vi "RFswitch2.vi"() -> ()   [LabVIEW 2013]
uses:
  Global 1.vi
panel:
  out "Ping result":u8 format="%x"
  out "Status":i32=1
  in  "RF Channel":u32=4 min=1 max=4 step=1
  out "Bytes Written 6":i32=5
  out "Bytes Read 6":i32
  out "Read Array 6":i32[](array[numeric])
  out "Write Array 6":i32[](array[numeric])=[5, 53, 6, 0, 0]
  out "Bytes Written 7":i32=5
  out "Bytes Read 7":i32
  out "Read Array 7":i32[](array[numeric])
  out "Write Array 7":i32[](array[numeric])=[5, 53, 7, 0, 0]
  out "Handle":u32=263961288
  in  "Controller Device Description":string="DLP-IO20"
  # "RF switch control panel"
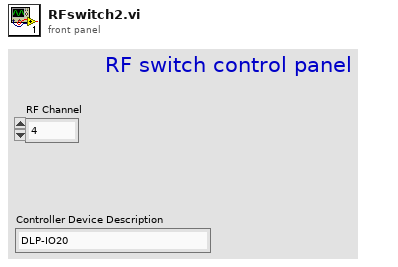
[diagram p1: front panel]
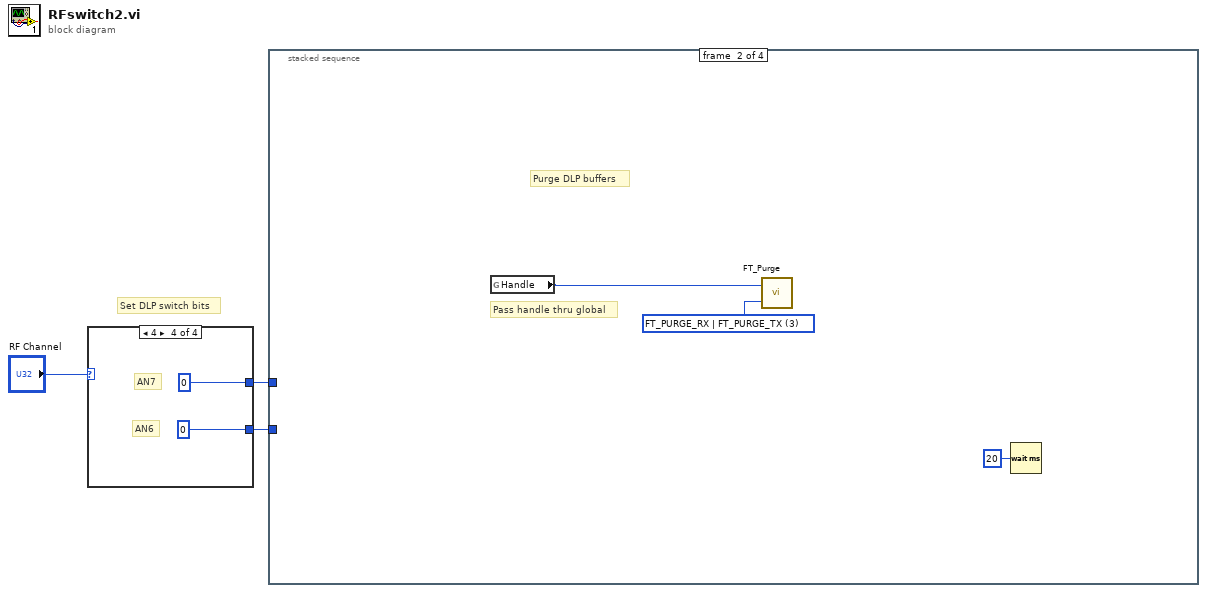
[diagram p0: block diagram]
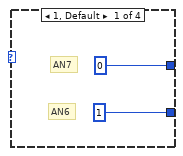
[diagram p2: hidden frame]
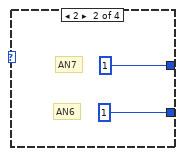
[diagram p3: hidden frame]
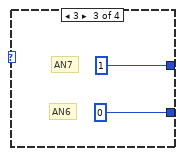
[diagram p4: hidden frame]
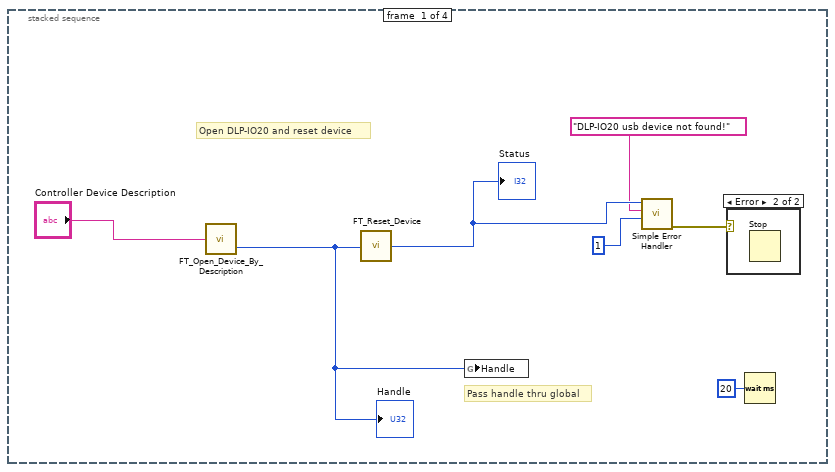
[diagram p5: hidden frame]
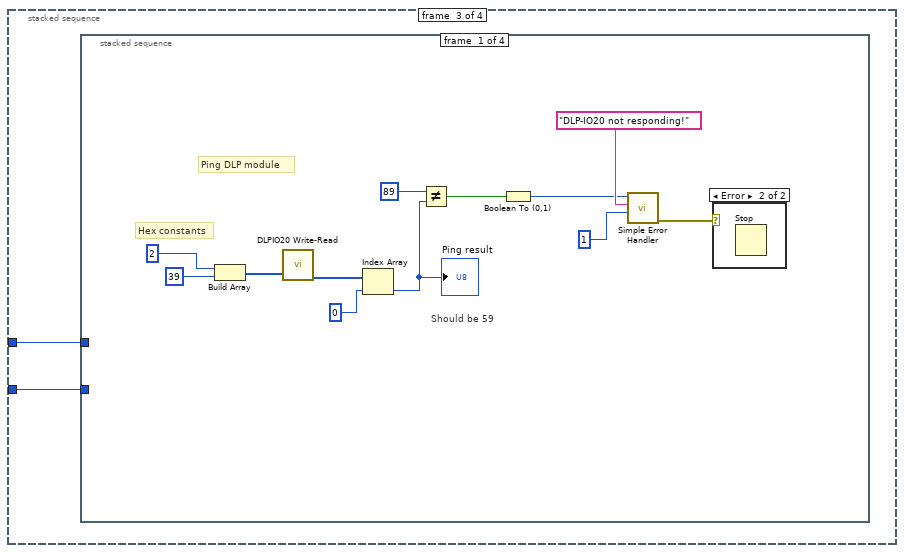
[diagram p7: hidden frame]
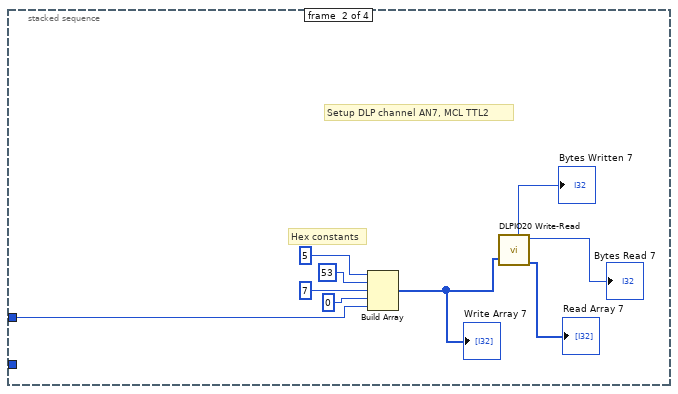
[diagram p9: hidden frame]
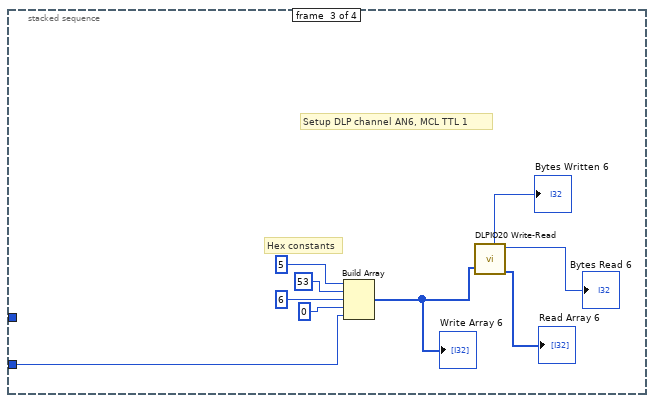
[diagram p10: hidden frame]
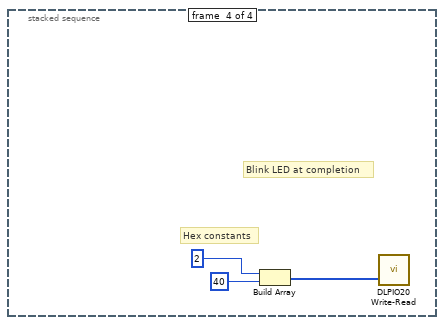
[diagram p11: hidden frame]
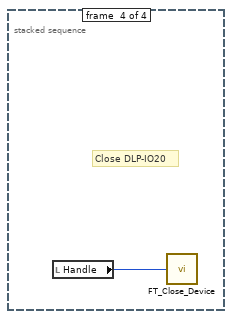
[diagram p12: hidden frame]
diagram:
  # "Set DLP switch bits"
  n1 = case shown="4" "RF Channel" {
    tunnel: [0 1 1 0] -> w2
    tunnel: [1 1 0 0] -> w1
    frame 1, Default {
      # "AN6"
      # "AN7"
    }
    frame 2 {
      # "AN6"
      # "AN7"
    }
    frame 3 {
      # "AN6"
      # "AN7"
    }
    frame 4 {
      # "AN6"
      # "AN7"
    }
  }
  n2 = stacked-sequence {
    tunnel: w2 -> [_ _ w23 _]
    tunnel: w1 -> [_ _ w22 _]
    frame #0 {
      # "Pass handle thru global"
      # "Open DLP-IO20 and reset device"
      n3 = call "FT_Open_Device_By_Description.vi"("Device Description"="Controller Device Description") -> ("Handle"=w16:u32)  [unwired: 1 out]
      "Handle" <- w16
      n4 = call "FT_Reset_Device.vi"("Handle"=w16) -> ("FT_Status"=w15:u32)
      "Status" <- w15
      n5 = global write "Global 1.vi" "Handle"(w16) -> ()
      n6 = call <vilib>:"Simple Error Handler.vi"("error code (no error:0)"=w15, "error source (\" \")"="DLP-IO20 usb device not found!", "type of dialog (OK msg:1)"=1) -> ("error out"=w12:errorcluster)  [unwired: 2 in, 4 out]
      n7 = case shown="Error" w12 {
        frame No Error {
        }
        frame Error {
          n8 = Stop() -> ()  [unwired: 1 in]
        }
      }
      n9 = Wait (ms)(milliseconds to wait=u32 20) -> ()  [unwired: 1 out]
    }
    frame #1 {
      w21 = u32 3 items=["FT_PURGE_RX"=1, "FT_PURGE_TX"=2, "FT_PURGE_RX | FT_PURGE_TX"=3] ("Purge Flags")
      # "Purge DLP buffers"
      # "Pass handle thru global"
      n10 = global read "Global 1.vi" "Handle"() -> (w20:u32)
      n11 = call "FT_Purge.vi"("Purge Flags"=w21, "Handle"=w20) -> ()  [unwired: 1 out]
      n12 = Wait (ms)(milliseconds to wait=u32 20) -> ()  [unwired: 1 out]
    }
    frame #2 {
      n13 = stacked-sequence {
        tunnel: w23 -> [_ w36 _ _]
        tunnel: w22 -> [_ _ w45 _]
        frame #0 {
          # "Should be 59"
          # "Ping DLP module"
          # "Hex constants"
          n14 = Build Array "Build Array"(u8 2, u8 39) -> (w33:u8[])
          n15 = call "DLPIO20 Write-Read.vi"("Write Buffer"=w33) -> ("Read Buffer Out"=w32:u8[])  [unwired: 3 in, 2 out]
          n16 = Index Array(array=w32, index=u8 0) -> (element=w29:u8)
          "Ping result" <- w29
          n17 = Not Equal?(x=u8 89, y=w29) -> (x != y?=w25:bool)
          n18 = Boolean To (0,1)(Boolean=w25) -> (0, 1=w24:i16)
          n19 = call <vilib>:"Simple Error Handler.vi"("error code (no error:0)"=w24, "error source (\" \")"="DLP-IO20 not responding!", "type of dialog (OK msg:1)"=1) -> ("error out"=w26:errorcluster)  [unwired: 2 in, 4 out]
          n20 = case shown="Error" w26 {
            frame No Error {
            }
            frame Error {
              n21 = Stop() -> ()  [unwired: 1 in]
            }
          }
        }
        frame #1 {
          # "Setup DLP channel AN7, MCL TTL2"
          # "Hex constants"
          n22 = Build Array "Build Array"(u8 5, u8 53, u8 7, u8 0, w36) -> (w39:i32[])
          "Write Array 7" <- w39
          n23 = call "DLPIO20 Write-Read.vi"("Write Buffer"=w39) -> ("Read Buffer Out"=→"Read Array 7":u8[], "Bytes Read"=→"Bytes Read 7":u32, "Bytes Written"=→"Bytes Written 7":u32)  [unwired: 3 in]
        }
        frame #2 {
          # "Setup DLP channel AN6, MCL TTL 1"
          # "Hex constants"
          n24 = Build Array "Build Array"(u8 5, u8 53, u8 6, u8 0, w45) -> (w48:i32[])
          "Write Array 6" <- w48
          n25 = call "DLPIO20 Write-Read.vi"("Write Buffer"=w48) -> ("Read Buffer Out"=→"Read Array 6":u8[], "Bytes Read"=→"Bytes Read 6":u32, "Bytes Written"=→"Bytes Written 6":u32)  [unwired: 3 in]
        }
        frame #3 {
          # "Blink LED at completion"
          # "Hex constants"
          n26 = Build Array "Build Array"(u8 2, u8 40) -> (w54:u8[])
          n27 = call "DLPIO20 Write-Read.vi"("Write Buffer"=w54) -> ()  [unwired: 3 in, 3 out]
        }
      }
    }
    frame #3 {
      # "Close DLP-IO20"
      n28 = local read "Handle"() -> (w57:u32)
      n29 = call "FT_Close_Device.vi"("Handle"=w57) -> ()  [unwired: 1 out]
    }
  }
